vi "ep04_digital_outputs.vi"() -> ()   [LabVIEW 2019]
panel:
  in  "LED0 Off":bool
  in  "LED0 On":bool
  in  "Toggle LED3":bool
  in  "stop":bool
  out "Service Status":bool
  out "Port Status":bool
  out "Information":string
  in  "Baud Rate":T1(ring)=enum."115200"
  in  "Port Id":T2(ring) caption="Port Name"
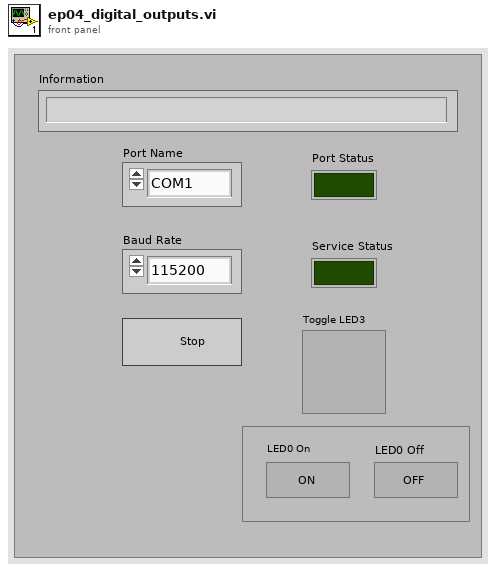
[diagram p1: front panel]
types:
  T1 = enum32{"300", "600", "1200", "2400", "4800", "9600", "14400", "19200", "28800", "38400", "56000", "57600", "115200", "128000", "256000"}
  T2 = enum8{"COM1", "COM2", "COM3", "COM4", "COM5", "COM6", "COM7", "COM8", "COM9", "COM10", "COM11", "COM12", "COM13", "COM14", "COM15", "COM16", "COM17", "COM18", "COM19", "COM20", "COM21", "COM22", "COM23", "COM24", "COM25", "COM26", "COM27", "COM28", "COM29", "COM30", "COM31", "COM32", "COM33", "COM34", "COM35", "COM36", "COM37", "COM38", "COM39", "COM40", "COM41", "COM42", "COM43", "COM44", "COM45", "COM46", "COM47", "COM48"}
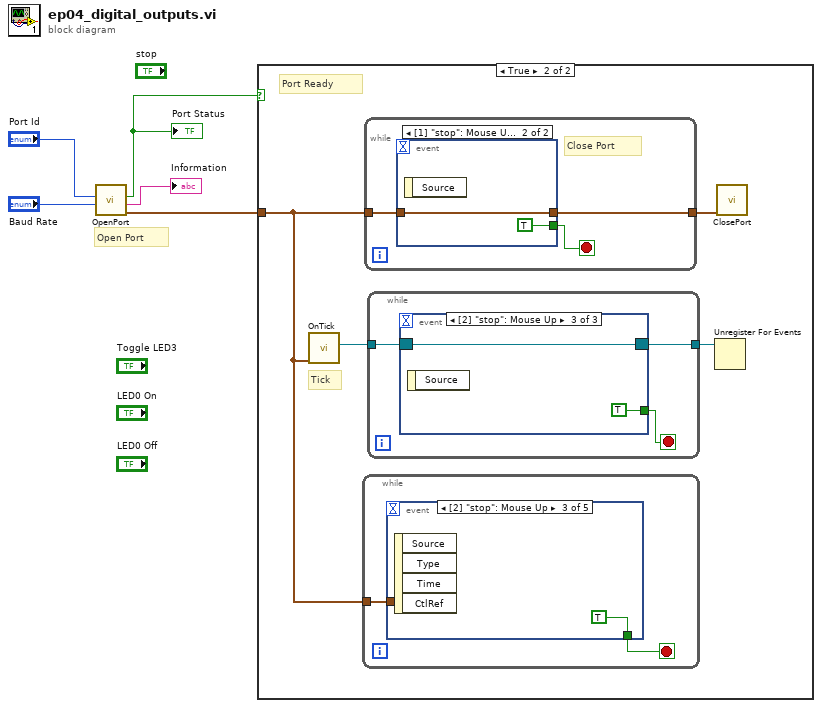
[diagram p0: block diagram]
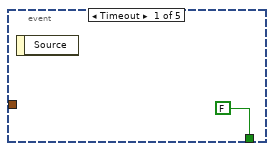
[diagram p3: hidden frame]
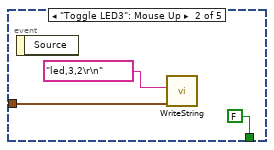
[diagram p4: hidden frame]
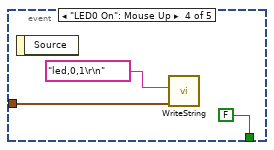
[diagram p5: hidden frame]
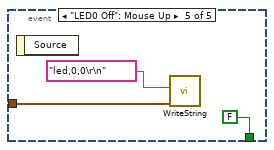
[diagram p6: hidden frame]
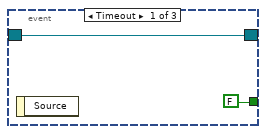
[diagram p7: hidden frame]
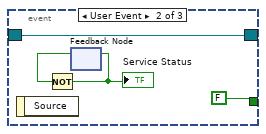
[diagram p8: hidden frame]
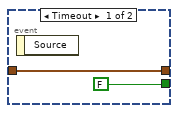
[diagram p9: hidden frame]
diagram:
  # "Open Port"
  n1 = call "OpenPort.vi"("Baud Rate Input"="Baud Rate", "Port Id Input"="Port Id") -> ("Uart Output"=w1:cluster{u64}, "Information"=→"Information":string, "Port Status"=w2:bool)  [unwired: 6 in, 1 out]
  "Port Status" <- w2
  n2 = case shown="True" w2 {
    tunnel: w1 -> [_ w6]
    frame False {
      # "Do nothing"
    }
    frame True {
      # "Tick"
      # "Port Ready"
      n3 = call "OnTick.vi"("Uart Input"=w6) -> ("On Tick Event"=w9:refnum<event-registration>)  [unwired: 8 in, 2 out]
      n4 = while {
        tunnel: w6 -> [w11]
        stop <- w10 stop-if-true
        n5 = event shown="[2] \"stop\": Mouse Up" {
          selector: _ -> [_ _ _ _ _]
          dyn-events: _ -> [_ _ _ _ _]
          timeout: _ -> [_ _ _ _ _]
          tunnel: w11 -> [_ w15 _ w18 w21]
          tunnel: [FALSE FALSE TRUE FALSE FALSE] -> w10
          event Timeout {
            n6 = event-data() -> ()  [unwired: 1 in, 1 out]
          }
          event "Toggle LED3": Mouse Up {
            n7 = event-data() -> ()  [unwired: 1 in, 1 out]
            n8 = call "WriteString.vi"("Uart Input"=w15, "String Data"="led,3,2\r\n") -> ()  [unwired: 7 in, 3 out]
          }
          event "stop": Mouse Up {
            n9 = event-data() -> ()  [unwired: 1 in, 4 out]
          }
          event "LED0 On": Mouse Up {
            n10 = event-data() -> ()  [unwired: 1 in, 1 out]
            n11 = call "WriteString.vi"("Uart Input"=w18, "String Data"="led,0,1\r\n") -> ()  [unwired: 7 in, 3 out]
          }
          event "LED0 Off": Mouse Up {
            n12 = event-data() -> ()  [unwired: 1 in, 1 out]
            n13 = call "WriteString.vi"("Uart Input"=w21, "String Data"="led,0,0\r\n") -> ()  [unwired: 7 in, 3 out]
          }
        }
      }
      n14 = while {
        tunnel: w6 -> [w35]
        tunnel: [w34] -> w7
        stop <- w36 stop-if-true
        # "Close Port"
        n15 = event shown="[1] \"stop\": Mouse Up" {
          selector: _ -> [_ _]
          dyn-events: _ -> [_ _]
          timeout: _ -> [_ _]
          tunnel: [FALSE TRUE] -> w36
          tunnel: w35 -> [w37 w39]
          tunnel: [w37 w39] -> w34
          event Timeout {
            n16 = event-data() -> ()  [unwired: 1 in, 1 out]
          }
          event "stop": Mouse Up {
            n17 = event-data() -> ()  [unwired: 1 in, 1 out]
          }
        }
      }
      n18 = while {
        tunnel: w9 -> [w24]
        tunnel: [w23] -> w8
        stop <- w25 stop-if-true
        n19 = event shown="[2] \"stop\": Mouse Up" {
          selector: w24 -> [w26 w28 w32]
          dyn-events: [w26 w28 w32] -> w23
          timeout: _ -> [_ _ _]
          tunnel: [FALSE FALSE TRUE] -> w25
          event Timeout {
            n20 = event-data() -> ()  [unwired: 1 in, 1 out]
          }
          event User Event {
            n21 = event-data() -> ()  [unwired: 1 in, 1 out]
            n22 = feedback #1() -> (w30:bool)  [unwired: 1 in]
            n23 = Not(x=w30) -> (.not. x?=w29:bool)
            "Service Status" <- w29
            n24 = feedback-in #1(w29) -> ()
          }
          event "stop": Mouse Up {
            n25 = event-data() -> ()  [unwired: 1 in, 1 out]
          }
        }
      }
      n26 = Unregister For Events(event registration refnum=w8) -> ()  [unwired: 1 in, 1 out]
      n27 = call "ClosePort.vi"("Uart Input"=w7) -> ()  [unwired: 9 in, 2 out]
    }
  }
